vi "MESADCGetTestDataEx.vi"(2 "barcode":string, 5 "错误输入（无错误）":errorcluster) -> (15 "布尔":bool, 16 "databuf":string, 18 "message":string, 19 "错误输出":errorcluster)   [LabVIEW 2014]
uses:
  dll/MESControldll.dll
panel:
  out "errbuf":string
  out "m_paramAVal":string
  out "PointGroup 2":string
  out "PointName 2":string
  out "userid 2":string
  out "result 2":i32
  out "POnum 1":i32
  out "result":i32
  # "2300013"
  # "447BBBCDFA60"
  # "MES:CHECK OK"
  # "1001594"
  # "0是代表OK，-1代表NG"
  # "计算机名"
  # "447BBBA1A0D0"
  # "MES:SN [EC82637A4880] \n不允许此测试 [F2]! 当前节点 [F1]"
  # "1001608"
  # "EC8263799B78\nSay{FAIL.wav}请维护规程 [整机维修] 的测试代码!"
  # "85353"
  # "OnMESADCGetTestDataEx(\"MACDATA\", (LPSTR)(LPCTSTR)m_scan_mac, \"\", \"\", \"\", databuf, errbuf);"
  # "获取MAC信息的表：MACDATA\n获取BOSASN的表：GETBOSA_SN"
  # "2300013\n18132D7F0694\n85174\nF6信息核对"
  # "2300013\n447BBBA12C40\n85197\nF6接口测试"
  # "2300013\nEC82637770B0\n85255\nF1信息写入"
  # "38E1AAC46018,C9F5CBB6,GC9F5CBB6,ZTEGC9F5CBB6,38E1AA,ZTEGC9F5CBB6,fx643,CMCC-U6QX,njrp629n,YE180220016187,"
  # "F650:\n1ssid:0C3747CEA600,C65DD431,GC65DD431,ZTEGC65DD431,0C3747,3D8330C3747CEA600,zwqpa,ChinaNet-SeF4,xnsxspr6,G1017J011893,\n2ssid:38E1AA14FF00,C65CC2C1,GC65CC2C1,ZTEGC65CC2C1,38E1AA,4086438E1AA14FF00,kpzjd,ChinaNet-Z5RL,z2ntvu6n,iTV-Z5RL,"
  # "F663:\n1ssid:4CABFC442A40,C9F6DA01,GC9F6DA01,ZTEGC9F6DA01,4CABFC,ZTEGC9F6DA01,eugr9,CMCC-76Kz,7grrcfa2,YC180300008186,\n2ssid:7C39531C7021,C9F2C308,GC9F2C308,ZTEGC9F2C308,7C3953,ZTEGC9F2C308,us6gy,CMCC-y9a9,g97yp3ty,YZ174800036588,"
  # "38E1AAC46018\n38E1AAC46010"
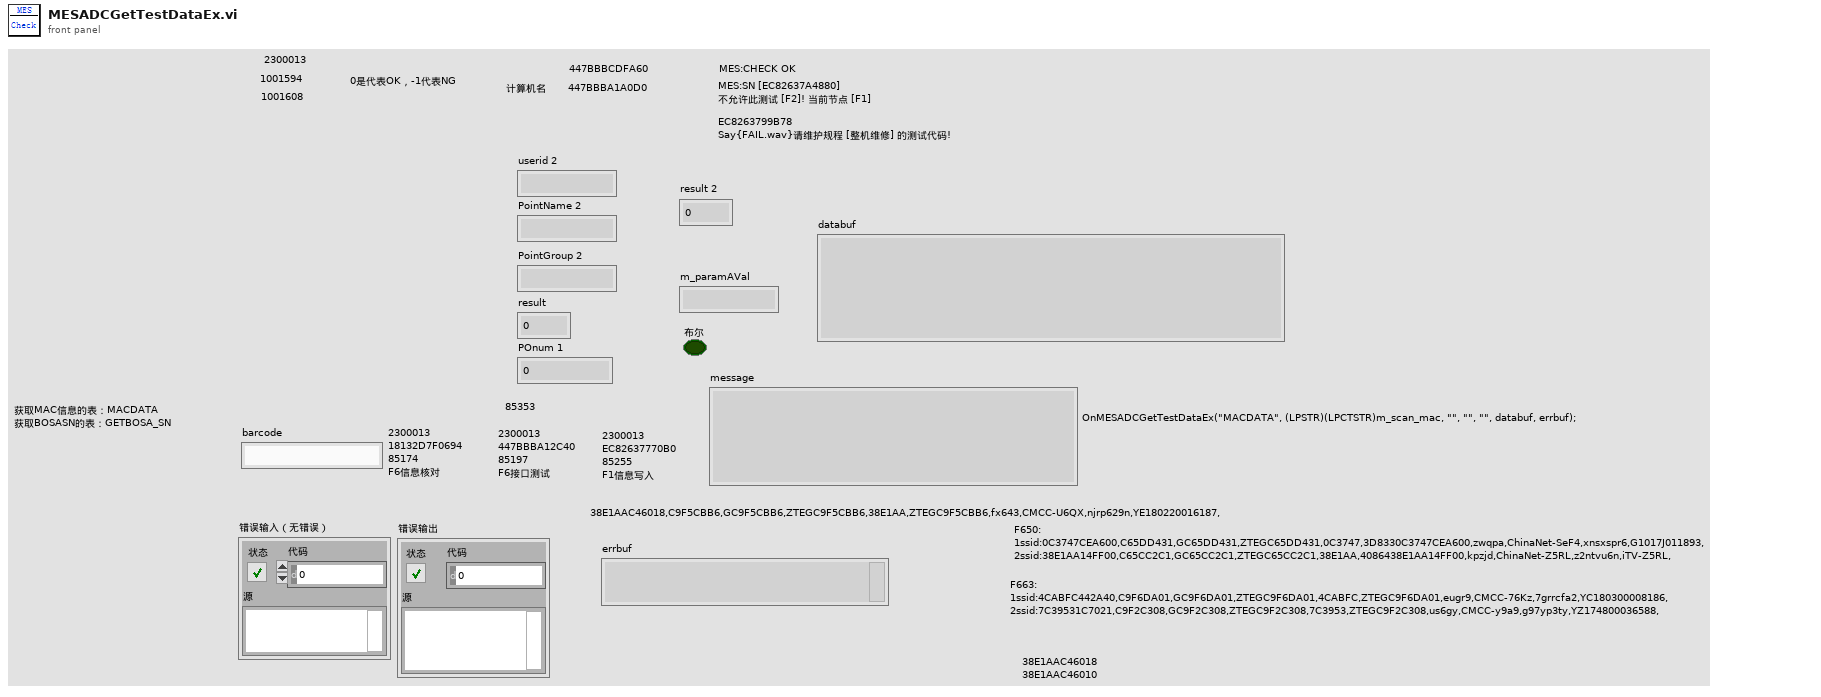
[diagram p1: front panel]
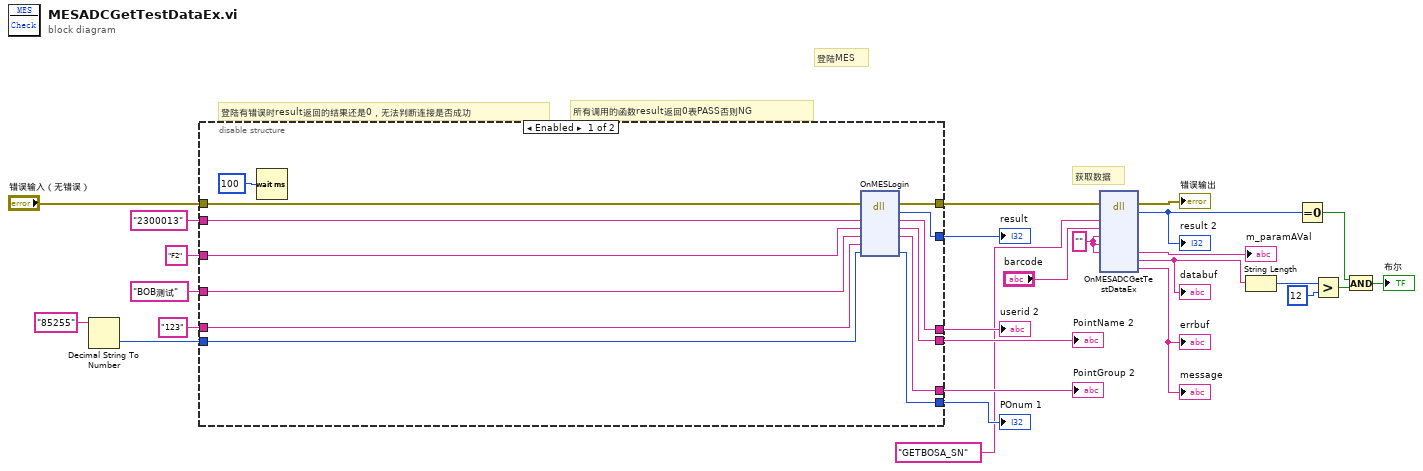
[diagram p0: block diagram]
diagram:
  w16 = ""
  # "登陆MES"
  # "获取数据"
  # "登陆有错误时result返回的结果还是0，无法判断连接是否成功"
  # "所有调用的函数result返回0表PASS否则NG"
  n1 = Decimal String To Number(string="85255") -> (number=w17:i32)  [unwired: 2 in, 1 out]
  n2 = disable-structure shown="Enabled" {
    disable-tunnel: "错误输入（无错误）" -> [w39 w40]
    disable-tunnel: [w38 _] -> w23
    disable-tunnel: [w37 _] -> w22
    disable-tunnel: [w36 _] -> w21
    disable-tunnel: [w35 _] -> w20
    disable-tunnel: [w34 _] -> w18
    disable-tunnel: "2300013" ("string") -> [w33 _]
    disable-tunnel: "BOB测试" ("string") -> [w32 _]
    disable-tunnel: "F2" ("string") -> [w31 _]
    disable-tunnel: "123" ("string") -> [w30 _]
    disable-tunnel: w17 -> [w29 _]
    disable-tunnel: [w28 w40] -> w1
    frame Enabled {
      n3 = Wait (ms)(milliseconds to wait=u32 100 ("等待时间（毫秒）")) -> ()  [unwired: 1 out]
      n4 = dll-call lib="PTH2Sabs D工作\tBOB软件\tBOB_25L95BOB_ZTE_GN25L95MESdllMESControldll.dll" fn="OnMESLogin"(error in=w39, "userid"=w33, "PointName"=w31, "PointGroup"=w32, "PointPlace"=w30, "EquipID"=w29) -> (error out=w28:errorcluster, "result"=w38:i32, "userid"=w37:string, "PointName"=w36:string, "PointGroup"=w35:string, "EquipID"=w34:i32)  [unwired: 3 in, 1 out]
    }
    frame Disabled {
    }
  }
  "result" <- w23
  "POnum 1" <- w18
  "userid 2" <- w22
  "PointName 2" <- w21
  "PointGroup 2" <- w20
  n5 = dll-call lib="PTH2Sabs D工作\tBOB软件\tBOB_25L95BOB_ZTE_GN25L95MESdllMESControldll.dll" fn="OnMESADCGetTestDataEx"(error in=w1, "data"="GETBOSA_SN" ("表名称"), "barcode"="barcode", "1"=w16, "2"=w16, "3"=w16) -> (error out=→"错误输出":errorcluster, "result"=w15:i32, "3"=→"m_paramAVal":string, "databuf"=w13:string, "errbuf"=→"message" →"errbuf":string)  [unwired: 8 in, 1 out]
  "databuf" <- w13
  "result 2" <- w15
  n6 = String Length(string=w13) -> (length=w12:i32)
  n7 = Equal To 0?(x=w15) -> (x = 0?=w10:bool)
  n8 = Greater?(x=w12, y=12) -> (0:w11:bool)
  n9 = And(x=w10, y=w11) -> (x .and. y?=→"布尔":bool)
